vi "Data Access.vi"(8 "error in (no error)":errorcluster, 10 "Data Access Handler":refnum<class "Data Access Handler.lvclass">, 11 "Flex Msg in":refnum<class "Nested Sequence Msg.lvclass">) -> (0 "error out":errorcluster, 3 "Flex Msg out":refnum<class "Nested Sequence Msg.lvclass">)   [LabVIEW 2020, in "Sequencer.lvlib" / "Nested Sequence Msg.lvclass"]
doc: "Expose class private data to the front panel while letting the Data Access Handler class act on the data."
uses:
  Nested Sequence Msg.lvclass
  C:/Current projects/WS/PPL/HDH.Actor Framework.Core.Msg.lvlibp/Flex Msg/Flex Msg.lvclass
  PPL/HDH.Actor Framework.Core.Msg.lvlibp/Flex Msg/Data Access Handlers/Data Access Handler/Data Access Handler.lvclass
  Controls/Ctl_SequenceNameArrayCluster.ctl
  Nested Sequence Msg.lvclass/Nested Sequence Msg.ctl
panel:
  in  "Sequence Name Array":T1
  in  "Cancel":bool
  in  "OK":bool
  # "If using override only non looping is supported"
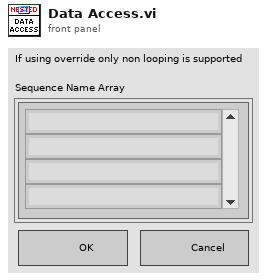
[diagram p1: front panel]
types:
  T1 = typedef "Sequencer.lvlib/Nested Sequence Msg.lvclass/Ctl_SequenceNameArrayCluster.ctl" = cluster{"Sequence Name Array":string[]}
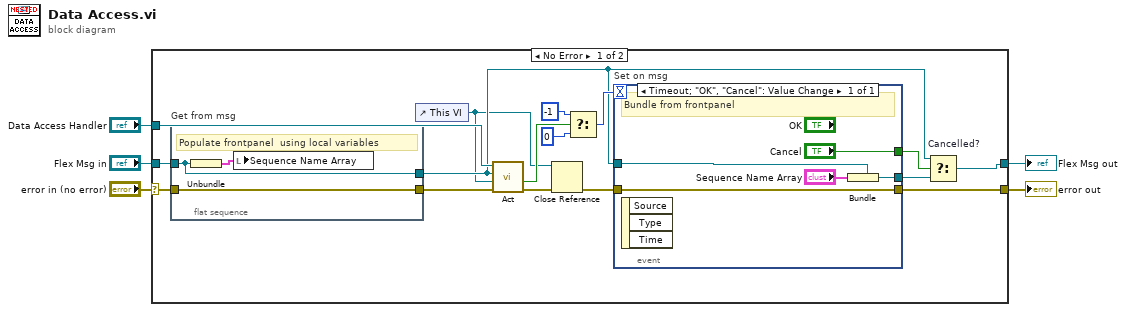
[diagram p0: block diagram]
diagram:
  n1 = case shown="No Error" "error in (no error)" {
    selector: "error in (no error)" -> [w21 w31]
    tunnel: [w14 w31] -> w4
    tunnel: [w9 w30] -> w2
    tunnel: "Flex Msg in" -> [w12 w30]
    tunnel: "Data Access Handler" -> [w20 _]
    frame No Error {
      n2 = flat-sequence "Get from msg" {
        tunnel: w21 -> [w29]
        tunnel: [w27] -> w7
        tunnel: w12 -> [w27]
        tunnel: [w29] -> w19
        frame #0 {
          # "Populate frontpanel  using local variables"
          n3 = Unbundle(w27) -> (w28:T1)
          n4 = local write "Sequence Name Array"(w28) -> ()
        }
      }
      n5 = control-ref of="This VI"() -> (w6:refnum<vi>)
      n6 = call-dynamic "Act.vi"("error in (no error)"=w19, "VI Refnum in"=w6, "Flex Msg type"=w7, "Data Access Handler in"=w20) -> ("error out"=w11:errorcluster, "Await user action?"=w18:bool)  [unwired: 5 in, 1 out]
      n7 = Close Reference(reference=w6, error in (no error)=w11) -> (error out=w13:errorcluster)
      n8 = Select(t=-1, s=w18, f=0 ("t")) -> (s? t:f=w15:i32)
      n9 = event "Set on msg" shown="[0] Timeout;  \"OK\", \"Cancel\": Value Change" {
        selector: _ -> [_]
        dyn-events: _ -> [_]
        timeout: w15 -> [_]
        tunnel: [w26] -> w14
        tunnel: w13 -> [w26]
        tunnel: ["Cancel"] -> w10
        tunnel: [w23] -> w8
        tunnel: w7 -> [w25]
        event Timeout; "OK", "Cancel": Value Change {
          # "Bundle from frontpanel"
          n10 = event-data() -> ()  [unwired: 1 in, 3 out]
          n11 = Bundle(cluster=w25, "Sequence Name Array") -> (w23:refnum<class "Nested Sequence Msg.lvclass">)
        }
      }
      n12 = Select "Cancelled?"(t=w7, s=w10, f=w8) -> (s? t:f=w9:refnum<class "Nested Sequence Msg.lvclass">)
    }
    frame Error {
    }
  }
  "error out" <- w4
  "Flex Msg out" <- w2
